vi "LDA_Analysis.vi"() -> (5 "Plug in titles":string[](array[string]), 7 "Plug in values":string[](array[string]))   [LabVIEW 2010]
uses:
  Controls/Save_Data.ctl
  Globals/LDA_meas_global_1.vi
  Globals/Plug_in_data_global.vi
  Globals/Meas_global.vi
  Globals/Constants_global.vi
  <vilib>/Analysis/NI_AALBase.lvlib
  <vilib>/gmath/NI_Gmath.lvlib
panel:
  out "XY Graph 2":T1(graph)
  in  "No of estimates output":i32=300
  out "Autocorrelation":cluster{dbl, dbl, dbl[]}[](graph)
  in  "Mode":enum16{"Spectra", "Autocorrelation"}(ring)
  in  "Separation Character":string="\t"
  in  "Precision":i16=2
  out "Ch names":string[](array[string])
  out "Number or Good blocks":i32
  out "Resampled block length":i32
  out "Resampling Frequency":dbl
  in  "Output Directory":path
  in  "File":T2=enum."Save Data"
  out "Frequency Spectrum":cluster{dbl, dbl, dbl[]}[](graph)
  # "You must have just these two indicators on the connector pane of the vi"
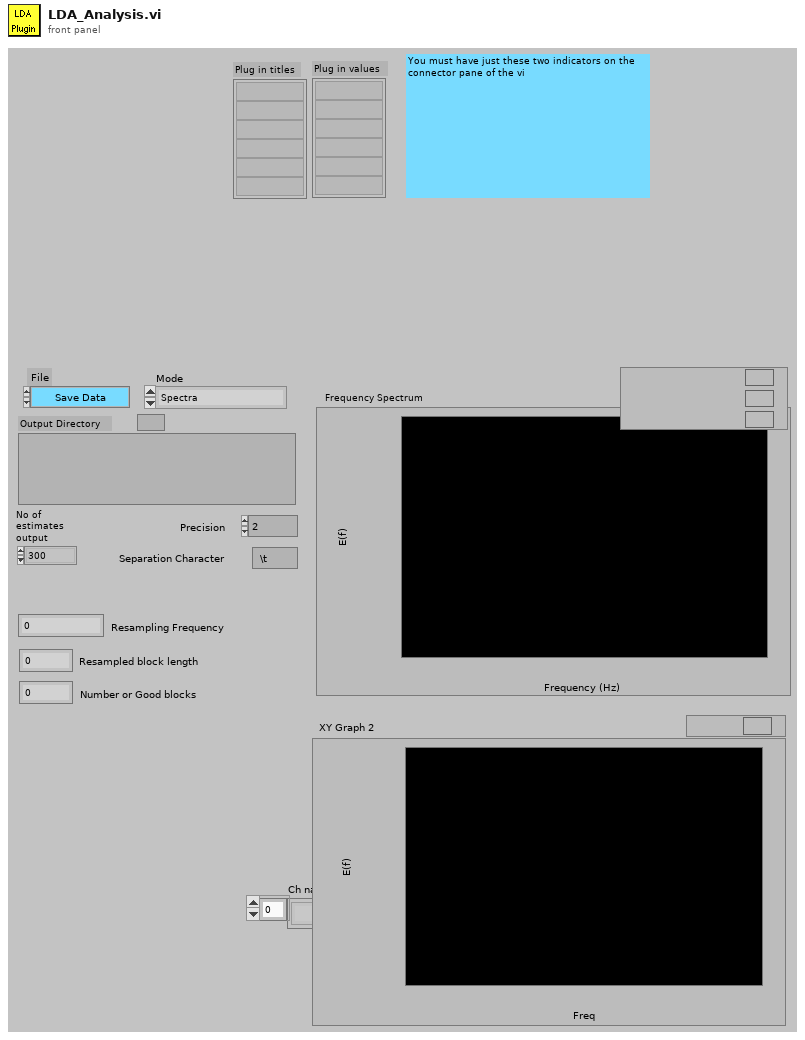
[diagram p1: front panel]
types:
  T1 = cluster{"Power Spectrum FFT {X} Frequency":dbl[], "Power Spectrum FFT {X}":dbl[]}
  T2 = typedef "Save_Data.ctl" = enum16{"Save No Data", "Save Data"}
  T3 = enum32{"existing file", "new file", "new or existing file", "existing dir", "new dir", "new or existing dir", "existing file (use LLBs)", "new file (use LLBs)", "new or existing file (use LLBs)", "new or existing file or directory (use LLBs)"}
  T4 = typedef "Analysis_info_cluster.ctl" = cluster{"Colour":u32, "Inst type":T5, "Inst name":string, "Symbol":string, "Code name":string, "Extra Info":string, "Inst Array":T6, "Index":i32, "Voltage Index":i32, "Extra Titles":string[], "Extra Values":string[]}
  T5 = typedef "Inst_type.ctl" = enum16{"Propeller anemometer", "Raw voltage", "Pressure Transducer", "Pitot-static tube", "Preston tube", "Hot wire", "Cross wire 1", "Cross wire 2", "Generic Linear", "Generic Polynomial", "Generic BackPoly", "Fast FID", "Thermocouple", "Cold wire", "Pulsed Wire", "LDA Vel", "LDA Tran time", "LDA Arr time"}
  T6 = typedef "Instrument_Array.ctl" = enum16{"PWA", "LDA", "Analogue"}
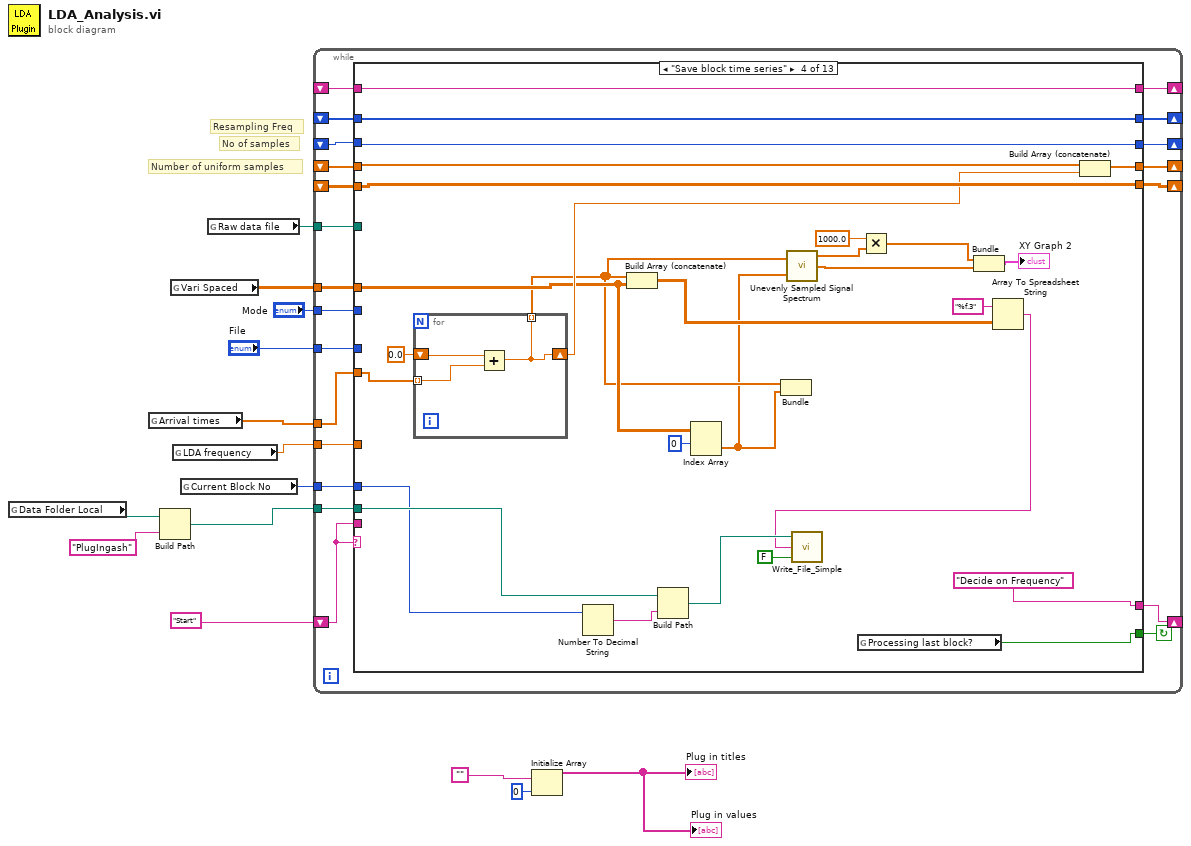
[diagram p0: block diagram]
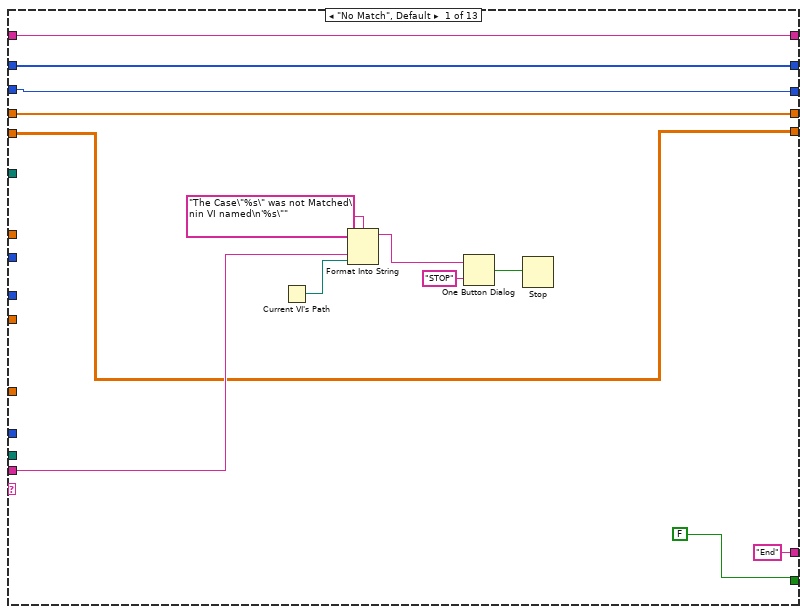
[diagram p2: hidden frame]
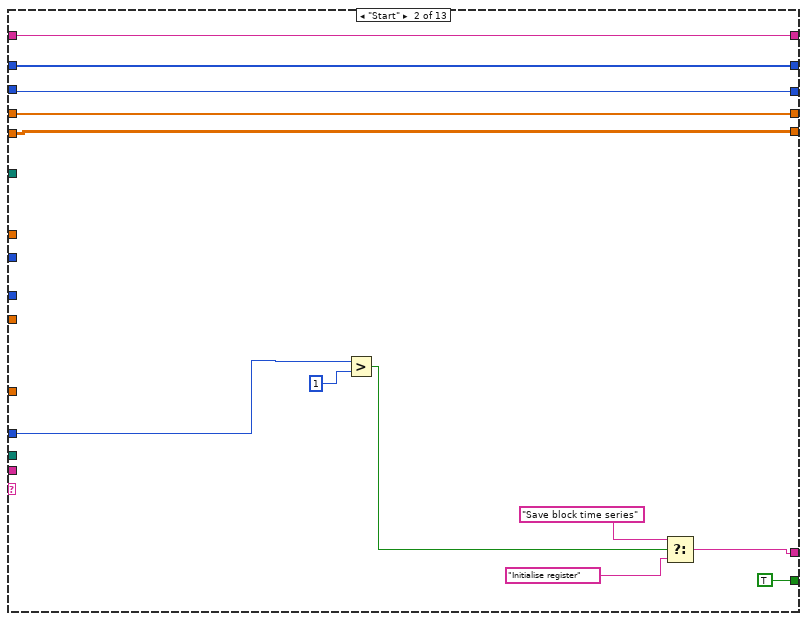
[diagram p3: hidden frame]
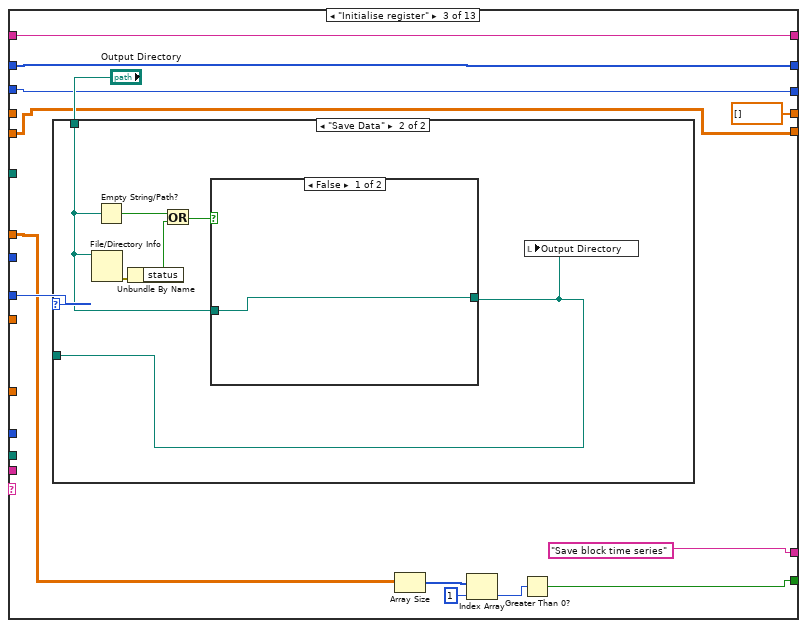
[diagram p4: hidden frame]
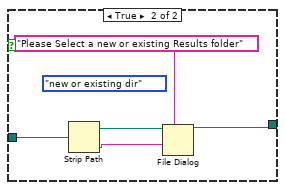
[diagram p6: hidden frame]
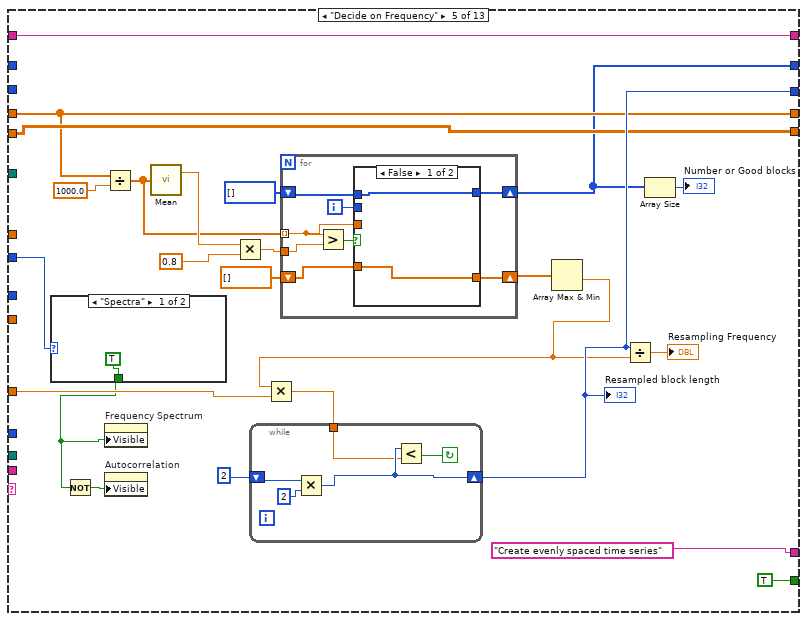
[diagram p7: hidden frame]
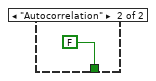
[diagram p8: hidden frame]
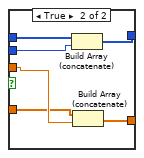
[diagram p9: hidden frame]
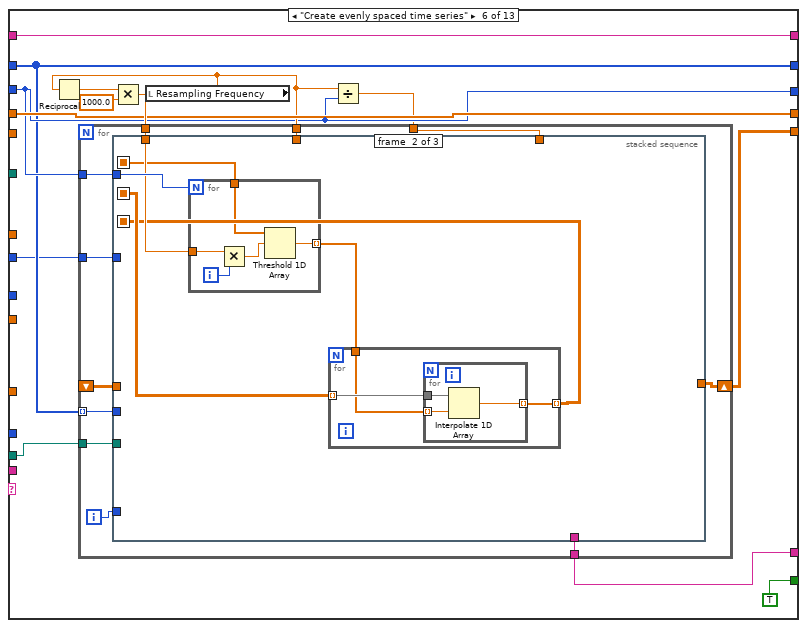
[diagram p10: hidden frame]
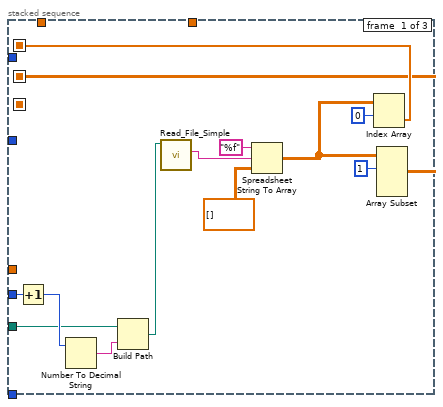
[diagram p11: hidden frame]
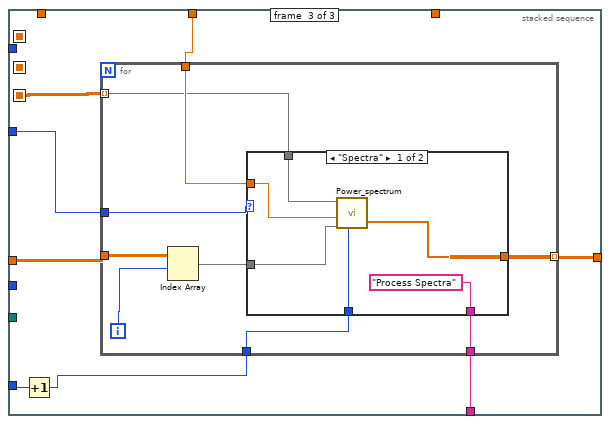
[diagram p12: hidden frame]
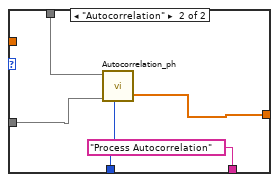
[diagram p13: hidden frame]
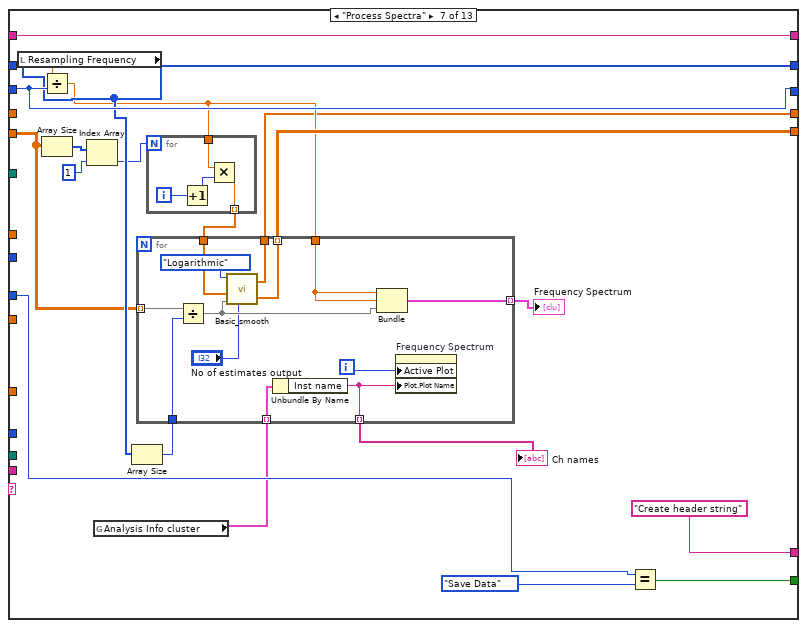
[diagram p14: hidden frame]
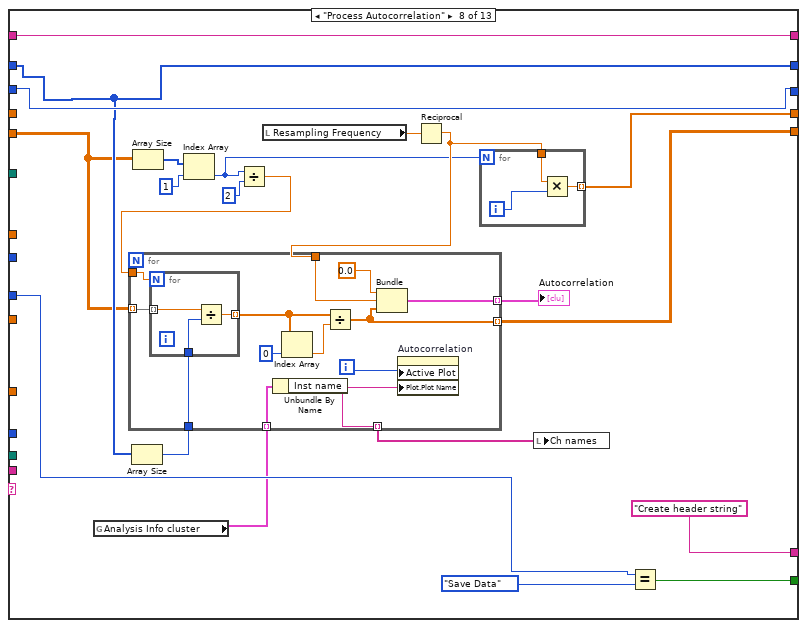
[diagram p15: hidden frame]
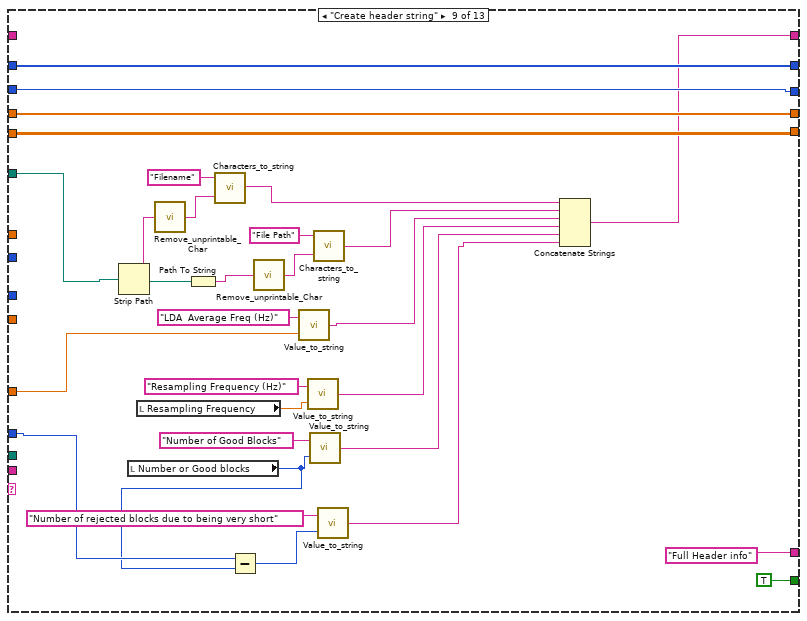
[diagram p16: hidden frame]
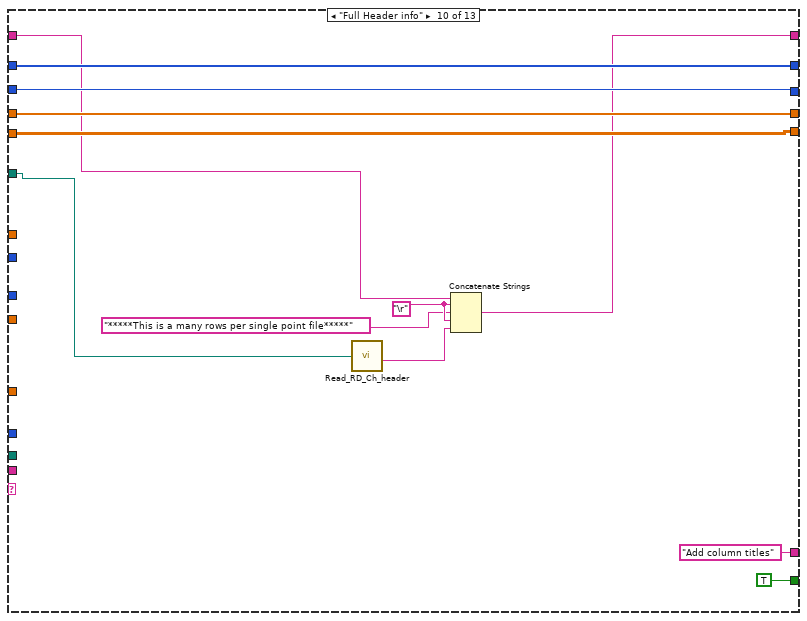
[diagram p17: hidden frame]
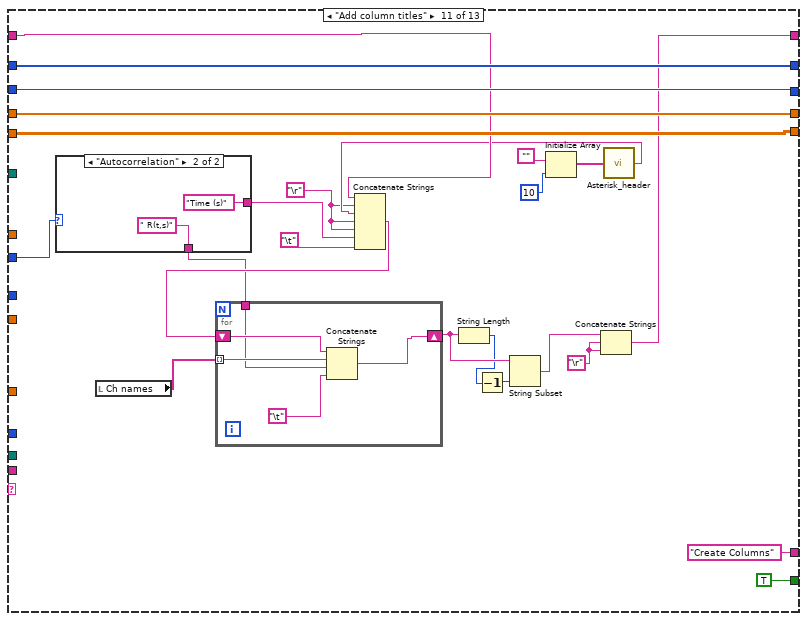
[diagram p18: hidden frame]
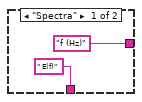
[diagram p19: hidden frame]
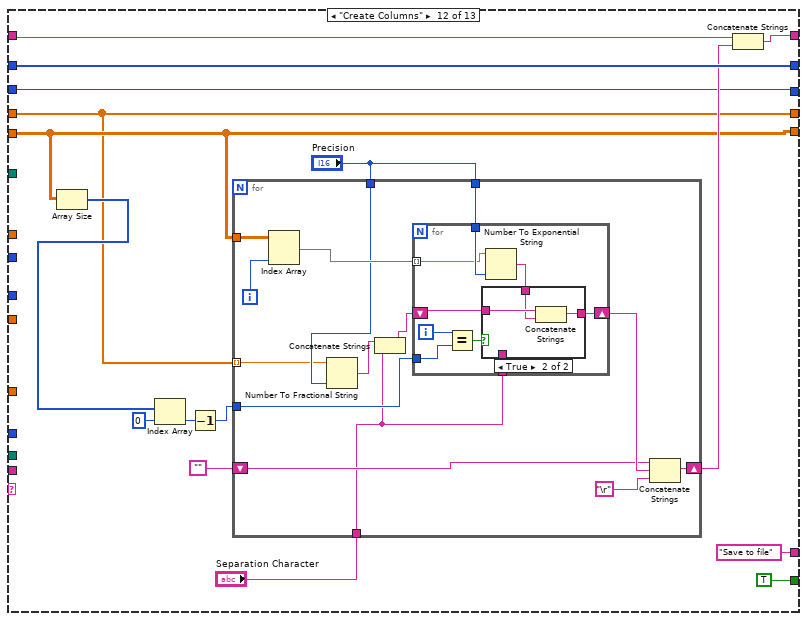
[diagram p20: hidden frame]
diagram:
  # "No of samples"
  # "Number of uniform samples"
  # "Resampling Freq"
  n1 = global read "Constants_global.vi" "Data Folder Local"() -> (w6:path)
  n2 = global read "LDA_meas_global_1.vi" "Arrival times"() -> (w12:dbl[])
  n3 = Build Path(base path=w6, name or relative path="PlugIngash") -> (appended path=w5:path)
  n4 = global read "Plug_in_data_global.vi" "Vari Spaced"() -> (w13:dbl[][])
  n5 = global read "Meas_global.vi" "LDA frequency"() -> (w2:dbl)
  n6 = global read "Meas_global.vi" "Current Block No"() -> (w8:i32)
  n7 = global read "Meas_global.vi" "Raw data file"() -> (w3:path)
  n8 = while {
    shift-left: "Start" -> [w35]
    shift-right: [w32] -> _
    tunnel: w13 -> [w34]
    tunnel: w12 -> [w33]
    shift-right: [w30] -> _
    shift-left: _ -> [w29]
    shift-right: [w28] -> _
    shift-left: _ -> [w27]
    tunnel: w8 -> [w26]
    tunnel: w5 -> [w25]
    shift-right: [w24] -> _
    shift-left: _ -> [w23]
    tunnel: "File" -> [w22]
    shift-right: [w21] -> _
    shift-left: _ -> [w20]
    tunnel: w3 -> [w19]
    tunnel: w2 -> [w18]
    shift-right: [w17] -> _
    shift-left: _ -> [w16]
    tunnel: "Mode" -> [w15]
    stop <- w31 continue-if-true
    n9 = case shown="\"Save block time series\"" w35 {
      tunnel: ["End" ("t") w55 "Save block time series" ("t") "Decide on Frequency" ("t") "Create evenly spaced time series" ("t") w165 "Create header string" "Create header string" "Full Header info" ("t") "Add column titles" ("t") "Create Columns" ("t") "Save to file" ("t") "End" ("t")] -> w32
      tunnel: w35 -> [w44 _ _ _ _ _ _ _ _ _ _ _ _]
      tunnel: w34 -> [_ _ w65 w94 _ _ _ _ _ _ _ _ _]
      tunnel: w33 -> [_ _ _ w101 _ _ _ _ _ _ _ _ _]
      tunnel: [FALSE TRUE w61 w106 TRUE TRUE ("Processing last block?") w261 w301 TRUE ("Processing last block?") TRUE ("Processing last block?") TRUE ("Processing last block?") TRUE ("Processing last block?") FALSE] -> w31
      tunnel: [w41 w51 w68 w102 w134 w174 w257 w295 w328 w363 w387 w405 _] -> w30
      tunnel: w29 -> [w41 w51 w68 w102 w134 _ w249 w292 w328 w363 w387 w405 _]
      tunnel: [w39 w54 dbl[] [] w104 w130 w173 w252 w286 w329 w364 w388 w400 w459] -> w28
      tunnel: w27 -> [w39 w54 _ w105 w130 w173 _ _ w329 w364 w388 w400 w459]
      tunnel: w26 -> [_ w53 _ w111 _ _ _ _ w337 _ _ _ _]
      tunnel: w25 -> [_ _ _ w112 _ w176 _ _ _ _ _ _ _]
      tunnel: [w40 w52 w69 w103 w135 w170 w264 w304 w330 w365 w389 w407 w460] -> w24
      tunnel: w23 -> [w40 w52 w69 w103 _ w170 w264 w304 w330 w365 w389 w407 w460]
      tunnel: w22 -> [_ _ w70 _ _ _ w262 w302 _ _ _ _ _]
      tunnel: [w38 w50 w67 w98 w124 w168 w256 w298 w331 w366 w390 w415 w458] -> w21
      tunnel: w20 -> [w38 w50 w67 w98 _ w168 w256 w298 w331 w366 w390 w415 w458]
      tunnel: w19 -> [_ _ _ _ _ _ _ _ w343 w356 _ _ w457]
      tunnel: w18 -> [_ _ _ _ w122 _ _ _ w340 _ _ _ _]
      tunnel: [w37 w49 w66 w97 w121 w167 w260 w300 w327 w355 w383 w411 w449] -> w17
      tunnel: w16 -> [w37 w49 w66 w97 w121 w167 w260 w300 _ w362 w377 w412 w449]
      tunnel: w15 -> [_ _ _ _ w120 w166 _ _ _ _ w380 _ w446]
      frame "No Match", Default {
        n10 = Current VI's Path() -> (path=w43:path)
        n11 = Format Into String(format string="The Case\"%s\" was not Matched\nin VI named\n'%s\"" ("Format String"), w44, w43) -> (resulting string=w47:string)  [unwired: 2 in, 1 out]
        n12 = One Button Dialog(message=w47, button name ("OK")="STOP") -> (true=w45:bool)
        n13 = Stop(stop? (T)=w45) -> ()
      }
      frame "Start" {
        n14 = Greater?(x=w53, y=1) -> (0:w57:bool)
        n15 = Select(t="Save block time series", s=w57, f="Initialise register") -> (s? t:f=w55:string)
      }
      frame "Initialise register" {
        n16 = case shown="\"Save Data\"" w70 {
          tunnel: [w74 w80] -> _
          tunnel: "Output Directory" -> [w74 w78]
          frame "Save No Data" {
          }
          frame "Save Data" {
            n17 = File/Directory Info(path=w78) -> (error out=w79:errorcluster)  [unwired: 1 in, 6 out]
            n18 = Empty String/Path?(string/path=w78) -> (empty?=w76:bool)
            n19 = Unbundle By Name(w79) -> ("status"=w77:bool)
            n20 = Or(x=w76, y=w77) -> (x .or. y?=w75:bool)
            n21 = case shown="False" w75 {
              tunnel: [w81 w86] -> w80
              tunnel: w78 -> [w81 w84]
              frame False {
              }
              frame True {
                (unwired) T3."new or existing dir" ("select mode (2)")
                n22 = Strip Path(path=w84) -> (stripped path=w83:path, name=w82:string)
                n23 = File Dialog(7:"Please Select a new or existing Results folder" ("prompt"), 9:w82, 11:w83) -> (3:w86:path)  [unwired: 1 in, 6 out]
              }
            }
            n24 = local write "Output Directory"(w80) -> ()
          }
        }
        n25 = Array Size(array=w65) -> (size(s)=w64:i32[])
        n26 = Index Array(array=w64, index=1) -> (element=w62:i32)
        n27 = Greater Than 0?(x=w62) -> (x > 0?=w61:bool)
      }
      frame "Save block time series" {
        n28 = for {
          shift-right: [w115] -> w99
          shift-left: 0.0 -> [w117]
          tunnel: w101 -> [w116] mode=indexing
          tunnel: [w115] -> w93 mode=indexing
          n29 = Add(x=w117, y=w116) -> (x+y=w115:dbl)
        }
        n30 = Number To Decimal String(number=w111) -> (decimal integer string=w110:string)  [unwired: 1 out]
        n31 = Build Array (concatenate)(w93, w94) -> (w96:dbl[][])
        n32 = Build Path(base path=w112, name or relative path=w110) -> (appended path=w109:path)
        n33 = Index Array(array=w94, index (row)=0) -> (element=w92:dbl[])  [unwired: 1 in]
        n34 = Bundle(w93, "Vari Spaced"=w92) -> ()  [unwired: 1 in, 1 out]
        n35 = call <vilib>:"Unevenly Sampled Signal Spectrum.vi"("XTime"=w93, "X"=w92) -> ("Power Spectrum FFT {X} Frequency"=w88:dbl[], "Power Spectrum FFT {X}"=w91:dbl[])  [unwired: 1 out]
        n36 = global read "Meas_global.vi" "Processing last block?"() -> (w106:bool)
        n37 = Multiply(x=1000.0, y=w88) -> (x*y=w87:dbl[])
        n38 = Bundle(w87, "Power Spectrum FFT {X}"=w91) -> (→"XY Graph 2":cluster{dbl[], "Power Spectrum FFT {X}":dbl[]})  [unwired: 1 in]
        n39 = Array To Spreadsheet String(array=w96, 3:"%f.3" ("format string")) -> (spreadsheet string=w108:string)  [unwired: 1 out]
        n40 = call "Write_File_Simple.vi"("append to file? (new file:F)"=FALSE, "character string"=w108, "file path"=w109) -> ()  [unwired: 2 out]
        n41 = Build Array (concatenate)(w105, w99) -> (w104:dbl[])
      }
      frame "Decide on Frequency" {
        n42 = case shown="\"Spectra\"" w120 {
          tunnel: [TRUE FALSE] -> w118
          frame "Spectra" {
          }
          frame "Autocorrelation" {
          }
        }
        n43 = Not(x=w118) -> (.not. x?=w119:bool)
        n44 = Divide(x=w130, y=1000.0) -> (x/y=w128:dbl[])
        n45 = property on="Frequency Spectrum" class="WFGraph (strict)"("Visible"=w118) -> ()  [unwired: 2 in, 2 out]
        n46 = property on="Autocorrelation" class="WFGraph (strict)"("Visible"=w119) -> ()  [unwired: 2 in, 2 out]
        n47 = call <vilib>:"Mean.vi"("X"=w128) -> ("mean"=w133:dbl)  [unwired: 1 out]
        n48 = Multiply(x=w133, y=0.8) -> (x*y=w131:dbl)
        n49 = for {
          tunnel: w128 -> [w146] mode=indexing
          tunnel: w131 -> [w151]
          shift-right: [w147] -> w124
          shift-left: i32[] [] -> [w148]
          shift-right: [w144] -> w126
          shift-left: dbl[] [] -> [w145]
          i -> [w149]
          n50 = Greater?(x=w146, y=w151) -> (0:w150:bool)
          n51 = case shown="False" w150 {
            tunnel: w149 -> [_ w159]
            tunnel: w148 -> [w153 w158]
            tunnel: [w153 w157] -> w147
            tunnel: w146 -> [_ w156]
            tunnel: w145 -> [w152 w155]
            tunnel: [w152 w154] -> w144
            frame False {
            }
            frame True {
              n52 = Build Array (concatenate)(w158, w159) -> (w157:i32[])
              n53 = Build Array (concatenate)(w155, w156) -> (w154:dbl[])
            }
          }
        }
        n54 = Array Max & Min(array=w126) -> (min value=w125:dbl)  [unwired: 3 out]
        n55 = Multiply(x=w125, y=w122) -> (x*y=w137:dbl)
        n56 = while {
          shift-right: [w162] -> w135
          shift-left: 2 -> [w164]
          tunnel: w137 -> [w161]
          stop <- w160 continue-if-true
          n57 = Multiply(x=w164, y=2) -> (x*y=w162:i32)
          n58 = Less?(x=w162, y=w161) -> (x < y?=w160:bool)
        }
        "Resampled block length" <- w135
        n59 = Divide(x=w135, y=w125) -> (x/y=→"Resampling Frequency":dbl)
        n60 = Array Size(array=w124) -> (size(s)=→"Number or Good blocks":i32)
      }
      frame "Create evenly spaced time series" {
        n61 = local read "Resampling Frequency"() -> (w171:dbl)
        n62 = Reciprocal(x=w171) -> (1/x=w177:dbl)
        n63 = Multiply(x=w177, y=1000.0) -> (x*y=w175:dbl)
        n64 = Divide(x=w171, y=w170) -> (x/y=w169:dbl)
        n65 = for {
          tunnel: w176 -> [w189]
          tunnel: w170 -> [w188]
          tunnel: w175 -> [w187]
          shift-right: [w185] -> w174
          shift-left: _ -> [w186]
          tunnel: w171 -> [w184]
          tunnel: w169 -> [w183]
          tunnel: w168 -> [w181] mode=indexing
          tunnel: w166 -> [w180]
          tunnel: [w179] -> w165
          i -> [w182]
          n66 = stacked-sequence {
            seq-local: [w195 _ _] -> [_ w206 _]
            seq-local: [w192 _ _] -> [_ w204 _]
            seq-local: [_ w203 _] -> [_ _ w227]
            tunnel: w182 -> [_ _ w223]
            tunnel: w189 -> [w200 _ _]
            tunnel: w188 -> [_ w208 _]
            tunnel: w187 -> [_ w207 _]
            tunnel: w186 -> [_ _ w226]
            tunnel: [_ _ w225] -> w185
            tunnel: w184 -> [_ _ w224]
            tunnel: w183 -> [_ _ _]
            tunnel: w181 -> [w190 _ _]
            tunnel: w180 -> [_ _ w221]
            tunnel: [_ _ w220] -> w179
            frame #0 {
              n67 = Increment(x=w190) -> (x+1=w201:i32)
              n68 = Number To Decimal String(number=w201) -> (decimal integer string=w202:string)  [unwired: 1 out]
              n69 = Build Path(base path=w200, name or relative path=w202) -> (appended path=w199:path)
              n70 = call "Read_File_Simple.vi"("Filename"=w199) -> ("string"=w198:string)  [unwired: 2 in, 7 out]
              n71 = Spreadsheet String To Array(format string="%f", spreadsheet string=w198, array type (2D Dbl)=dbl[][] []) -> (array=w194:dbl[][])  [unwired: 1 out]
              n72 = Index Array(array=w194, index (row)=0) -> (element=w195:dbl[])  [unwired: 1 in]
              n73 = Array Subset(array=w194, index (row)=1 ("index")) -> (w192:dbl[][])  [unwired: 3 in]
            }
            frame #1 {
              n74 = for {
                N: w208 -> [_]
                tunnel: w207 -> [w218]
                tunnel: w206 -> [w216]
                tunnel: [w215] -> w205 mode=indexing
                i -> [w219]
                n75 = Multiply(x=w218, y=w219) -> (x*y=w217:dbl)
                n76 = Threshold 1D Array(2:w217, 3:w216) -> (0:w215:dbl)  [unwired: 1 out]
              }
              n77 = for {
                tunnel: [w211] -> w203 mode=indexing
                tunnel: w205 -> [w209]
                tunnel: w204 -> [w210] mode=indexing
                n78 = for {
                  tunnel: w210 -> [w214]
                  tunnel: w209 -> [w213] mode=indexing
                  tunnel: [w212] -> w211 mode=indexing
                  n79 = Interpolate 1D Array(1:w213, 2:w214) -> (0:w212:dbl)
                }
              }
            }
            frame #2 {
              n80 = Increment(x=w223) -> (x+1=w222:i32)
              n81 = for {
                tunnel: w227 -> [w232] mode=indexing
                tunnel: [w231] -> w225 mode=indexing
                tunnel: w226 -> [w236]
                tunnel: w224 -> [w233]
                tunnel: w222 -> [w230]
                tunnel: w221 -> [w229]
                tunnel: [w228] -> w220
                i -> [w234]
                n82 = Index Array(array=w236, index (row)=w234) -> (element=w235:dbl[])  [unwired: 1 in]
                n83 = case shown="\"Spectra\"" w229 {
                  tunnel: w235 -> [w242 w246]
                  tunnel: w233 -> [w241 _]
                  tunnel: w232 -> [w240 w247]
                  tunnel: [w239 w245] -> w231
                  tunnel: w230 -> [w238 w244]
                  tunnel: ["Process Spectra" ("t") "Process Autocorrelation" ("t")] -> w228
                  frame "Spectra" {
                    n84 = call "Power_spectrum.vi"("U"=w240, "Sampling frequency"=w241, "Spectrum input array"=w242, "Block No"=w238) -> ("Spectrum output array"=w239:dbl[])  [unwired: 1 in, 1 out]
                  }
                  frame "Autocorrelation" {
                    n85 = call "Autocorrelation_ph.vi"("X"=w247, "Autocorrelation of X"=w246, "Block No"=w244) -> ("Autocorrelation of X"=w245:dbl[])  [unwired: 2 in, 1 out]
                  }
                }
              }
            }
          }
        }
      }
      frame "Process Spectra" {
        (unwired) FALSE
        n86 = local read "Resampling Frequency"() -> (w265:dbl)
        n87 = Divide(x=w265, y=w264) -> (x/y=w254:dbl)
        n88 = Array Size(array=w249) -> (size(s)=w251:i32[])
        n89 = Index Array(array=w251, index=1) -> (element=w248:i32)
        n90 = global read "Meas_global.vi" "Analysis Info cluster"() -> (w258:T4[])
        n91 = Array Size(array=w256) -> (size(s)=w255:i32)
        n92 = for {
          N: w248 -> [_]
          tunnel: w254 -> [w269]
          tunnel: [w268] -> w253 mode=indexing
          i -> [w271]
          n93 = Increment(x=w271) -> (x+1=w270:i32)
          n94 = Multiply(x=w269, y=w270) -> (x*y=w268:dbl)
        }
        n95 = for {
          tunnel: w254 -> [w284]
          tunnel: w249 -> [w283] mode=indexing
          tunnel: w255 -> [w282]
          tunnel: [w281] -> w266 mode=indexing
          tunnel: w258 -> [w279] mode=indexing
          tunnel: [w278] -> w259 mode=indexing
          tunnel: [w273] -> w257 mode=indexing
          tunnel: w253 -> [w276]
          tunnel: [w272] -> w252
          i -> [w280]
          n96 = Divide(x=w283, y=w282) -> (x/y=w277:dbl[])
          n97 = call "Basic_smooth.vi"("Smoothing"=enum16{"Linear", "Logarithmic"}."Logarithmic", "X array in"=w276, "Y array in"=w277, "No of estimates output"="No of estimates output") -> ("X array Out"=w272:dbl[], "Y array Out"=w273:dbl[])  [unwired: 1 out]
          n98 = Unbundle By Name(w279) -> ("Inst name"=w278:string)
          n99 = Bundle(w284, w284, w277) -> (w281:cluster{dbl, dbl, dbl[]})  [unwired: 1 out]
          n100 = property on="Frequency Spectrum" class="WFGraph (strict)"("Active Plot"=w280, "Plot.Plot Name"=w278) -> ()  [unwired: 2 in, 2 out]
        }
        "Frequency Spectrum" <- w266
        "Ch names" <- w259
        n101 = Equal?(x=w262, y=Save_Data."Save Data" ("File")) -> (x = y?=w261:bool)
      }
      frame "Process Autocorrelation" {
        (unwired) FALSE
        n102 = global read "Meas_global.vi" "Analysis Info cluster"() -> (w299:T4[])
        n103 = Array Size(array=w298) -> (size(s)=w297:i32)
        n104 = Array Size(array=w292) -> (size(s)=w291:i32[])
        n105 = Index Array(array=w291, index=1) -> (element=w285:i32)
        n106 = Divide(x=w285, y=2) -> (x/y=w288:dbl)
        n107 = local read "Resampling Frequency"() -> (w296:dbl)
        n108 = Reciprocal(x=w296) -> (1/x=w287:dbl)
        n109 = for {
          tunnel: w287 -> [w321]
          tunnel: w292 -> [w320] mode=indexing
          tunnel: w297 -> [w319]
          tunnel: [w318] -> w293 mode=indexing
          tunnel: w299 -> [w317] mode=indexing
          tunnel: [w312] -> w295 mode=indexing
          tunnel: [w310] -> w294 mode=indexing
          tunnel: w288 -> [w309]
          i -> [w311]
          n110 = for {
            N: w309 -> [_]
            tunnel: w320 -> [w324] mode=indexing
            tunnel: w319 -> [w323]
            tunnel: [w322] -> w314 mode=indexing
            n111 = Divide(x=w324, y=w323) -> (x/y=w322:dbl)
          }
          n112 = Unbundle By Name(w317) -> ("Inst name"=w310:string)
          n113 = Index Array(array=w314, index=0) -> (element=w313:dbl)
          n114 = Divide(x=w314, y=w313) -> (x/y=w312:dbl[])
          n115 = Bundle(0.0, w321, w312) -> (w318:cluster{dbl, dbl, dbl[]})  [unwired: 1 out]
          n116 = property on="Autocorrelation" class="WFGraph (strict)"("Active Plot"=w311, "Plot.Plot Name"=w310) -> ()  [unwired: 2 in, 2 out]
        }
        "Autocorrelation" <- w293
        n117 = for {
          N: w285 -> [_]
          tunnel: w287 -> [w308]
          tunnel: [w306] -> w286 mode=indexing
          i -> [w307]
          n118 = Multiply(x=w308, y=w307) -> (x*y=w306:dbl)
        }
        n119 = local write "Ch names"(w294) -> ()
        n120 = Equal?(x=w302, y=Save_Data."Save Data" ("File")) -> (x = y?=w301:bool)
      }
      frame "Create header string" {
        n121 = Strip Path(path=w343) -> (stripped path=w347:path, name=w351:string)
        n122 = local read "Number or Good blocks"() -> (w336:i32)
        n123 = local read "Resampling Frequency"() -> (w339:dbl)
        n124 = call "Remove_unprintable_Char.vi"("Input String"=w351) -> ("Output String"=w350:string)
        n125 = Path To String(path=w347) -> (string=w346:string)
        n126 = call "Characters_to_string.vi"("Characters to write"=w350, "Label for characters"="Filename") -> ("Output string"=w345:string)
        n127 = Subtract(x=w337, y=w336) -> (x-y=w335:i32)
        n128 = call "Remove_unprintable_Char.vi"("Input String"=w346) -> ("Output String"=w349:string)
        n129 = call "Value_to_string.vi"("Value"=w340, "Label for value"="LDA  Average Freq (Hz)") -> ("Output string"=w354:string)  [unwired: 1 in]
        n130 = call "Value_to_string.vi"("Value"=w339, "Label for value"="Resampling Frequency (Hz)") -> ("Output string"=w334:string)  [unwired: 1 in]
        n131 = call "Value_to_string.vi"("Value"=w336, "Label for value"="Number of Good Blocks") -> ("Output string"=w333:string)  [unwired: 1 in]
        n132 = call "Characters_to_string.vi"("Characters to write"=w349, "Label for characters"="File Path") -> ("Output string"=w344:string)
        n133 = call "Value_to_string.vi"("Value"=w335, "Label for value"="Number of rejected blocks due to being very short") -> ("Output string"=w332:string)  [unwired: 1 in]
        n134 = Concatenate Strings(w345, w344, w354, w334, w333, w332) -> (w327:string)
      }
      frame "Full Header info" {
        w359 = "\r"
        n135 = call "Read_RD_Ch_header.vi"("Raw data file"=w356) -> ("Ch string"=w357:string)  [unwired: 3 out]
        n136 = Concatenate Strings(w362, w359, "*****This is a many rows per single point file*****", w359, w357) -> (w355:string)
      }
      frame "Add column titles" {
        w371 = "\r"
        w372 = "\r"
        n137 = case shown="\"Autocorrelation\"" w380 {
          tunnel: ["f (Hz)" "Time (s)"] -> w379
          tunnel: [" E(f)" " R(t,s)"] -> w378
          frame "Spectra" {
          }
          frame "Autocorrelation" {
          }
        }
        n138 = local read "Ch names"() -> (w385:string[])
        n139 = Initialize Array("", 10) -> (w376:string[])
        n140 = call "Asterisk_header.vi"("Channel names"=w376) -> ("Header string"=w373:string)
        n141 = Concatenate Strings(w377, w371, w373, w371, w371, w379, "\t") -> (w384:string)
        n142 = for {
          shift-right: [w396] -> w370
          shift-left: w384 -> [w398]
          tunnel: w385 -> [w399] mode=indexing
          tunnel: w378 -> [w395]
          n143 = Concatenate Strings(w398, w399, w395, "\t") -> (w396:string)
        }
        n144 = String Length(string=w370) -> (length=w367:i32)
        n145 = Decrement(x=w367) -> (x-1=w368:i32)
        n146 = String Subset(string=w370, length (rest)=w368) -> (substring=w369:string)  [unwired: 1 out]
        n147 = Concatenate Strings(w369, w372, w372) -> (w383:string)
      }
      frame "Create Columns" {
        n148 = Array Size(array=w405) -> (size(s)=w403:i32[])
        n149 = Index Array(array=w403, index=0) -> (element=w402:i32)
        n150 = Decrement(x=w402) -> (x-1=w401:i32)
        n151 = for {
          shift-right: [w429] -> w410
          shift-left: "" -> [w424]
          tunnel: "Separation Character" -> [w417]
          tunnel: w405 -> [w427]
          tunnel: w401 -> [w423]
          tunnel: "Precision" -> [w421]
          tunnel: "Precision" -> [w420]
          tunnel: w400 -> [w416] mode=indexing
          i -> [w422]
          n152 = Index Array(array=w427, index (col)=w422) -> (element=w426:dbl[])  [unwired: 1 in]
          n153 = Number To Fractional String(number=w416, precision (6)=w420) -> (F-format string=w419:string)  [unwired: 2 out]
          n154 = Concatenate Strings(w419, w417) -> (w418:string)
          n155 = for {
            shift-right: [w436] -> w425
            shift-left: w418 -> [w438]
            tunnel: w417 -> [w435]
            tunnel: w426 -> [w430] mode=indexing
            tunnel: w423 -> [w433]
            tunnel: w421 -> [w431]
            i -> [w434]
            n156 = Equal?(x=w434, y=w433) -> (x = y?=w432:bool)
            n157 = Number To Exponential String(number=w430, precision (6)=w431) -> (E-format string=w437:string)  [unwired: 2 out]
            n158 = case shown="True" w432 {
              tunnel: w438 -> [w442 w445]
              tunnel: w437 -> [w441 w444]
              tunnel: [w440 w443] -> w436
              tunnel: w435 -> [w439 _]
              frame False {
                n159 = Concatenate Strings(w442, w441, w439) -> (w440:string)
              }
              frame True {
                n160 = Concatenate Strings(w445, w444) -> (w443:string)
              }
            }
          }
          n161 = Concatenate Strings(w424, w425, "\r") -> (w429:string)
        }
        n162 = Concatenate Strings(w412, w410) -> (w411:string)
      }
      frame "Save to file" {
        w451 = TRUE  # advisory dialog? (display:T)
        n163 = case shown="\"Autocorrelation\"" w446 {
          tunnel: ["Spec_" ("string") "Auto_" ("string")] -> w447
          frame "Spectra" {
          }
          frame "Autocorrelation" {
          }
        }
        n164 = Strip Path(path=w457) -> (name=w455:string)  [unwired: 1 out]
        n165 = local read "Output Directory"() -> (w456:path)
        n166 = Concatenate Strings(w447, w455) -> (w454:string)
        n167 = Build Path(base path=w456, name or relative path=w454) -> (appended path=w453:path)
        n168 = call "Create_directory_path.vi"("Path name"=w453) -> ("Path name Out"=w452:path)
        n169 = call "Write_Characters_To_File.vi"("file path (dialog if empty)"=w452, "advisory dialog? (display:T)"=w451, "character string"=w449, "append to file? (new file:F)"=FALSE) -> ()  [unwired: 1 in, 4 out]
      }
    }
  }
  n170 = Initialize Array("", 0) -> (→"Plug in values" →"Plug in titles":string[])
